vi "makeNames.vi"(11 "Strings":string[](array[string])) -> (3 "Names":string[](array[string]))   [LabVIEW 2014]
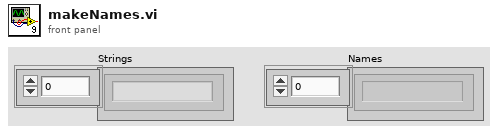
[diagram p1: front panel]
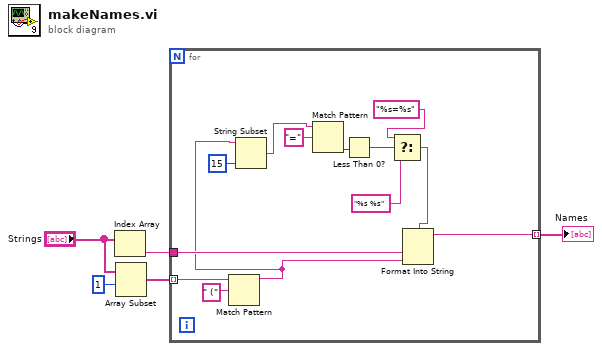
[diagram p0: block diagram]
diagram:
  n1 = Index Array(array="Strings") -> (element=w1:string)  [unwired: 1 in]
  n2 = Array Subset(array="Strings", index=1) -> (w2:string[])  [unwired: 1 in]
  n3 = for {
    tunnel: w2 -> [w17] mode=indexing
    tunnel: [w15] -> w4 mode=indexing
    tunnel: w1 -> [w16]
    n4 = Match Pattern(string=w17, regular expression=" (") -> (before substring=w11:string)  [unwired: 4 out]
    n5 = String Subset(string=w11, length (rest)=15 ("length (rest)")) -> (substring=w10:string)  [unwired: 1 in]
    n6 = Match Pattern(string=w10, regular expression="=") -> (offset past match=w13:i32)  [unwired: 1 in, 3 out]
    n7 = Less Than 0?(x=w13) -> (x < 0?=w9:bool)
    n8 = Select(t="%s=%s" ("format string"), s=w9, f="%s %s" ("Format String")) -> (s? t:f=w7:string)
    n9 = Format Into String(format string=w7, w16, w11) -> (resulting string=w15:string)  [unwired: 2 in, 1 out]
  }
  "Names" <- w4
